vi "SensorcolorV2.vi"() -> ()   [LabVIEW 2017]
panel:
  in  "Guardar en:":path
  out "Sin Filtro":dbl format="%.2f"
  out "Azul":dbl
  out "Verde":dbl format="%.2f"
  out "Rojo":dbl format="%.2f"
  in  "Frecuencia 1":bool=TRUE
  in  "Frecuencia 2":bool
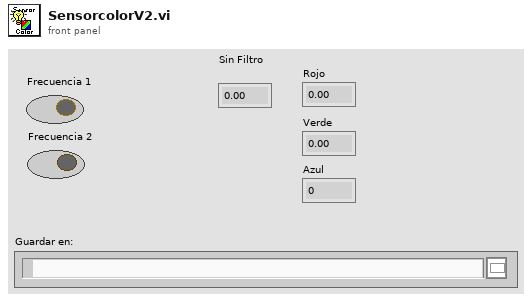
[diagram p1: front panel]
types:
  T1 = enum16{"open", "open or create", "create or replace", "create", "open (read-only)"}
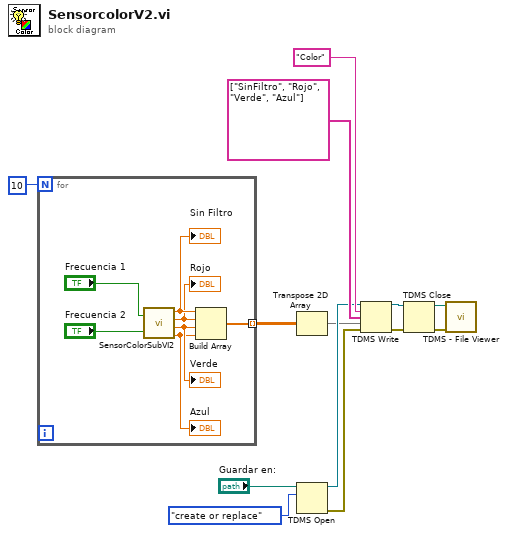
[diagram p0: block diagram]
diagram:
  n1 = for {
    N: 10 -> [_]
    tunnel: [w20] -> w4 mode=indexing
    n2 = call "SensorColorSubVI2.vi"("Frecuencia 1"="Frecuencia 1", "Frecuencia in"="Frecuencia 2") -> ("Sin Filtro"=w17:dbl, "Rojo"=w16:dbl, "Verde"=w15:dbl, "Azul"=w14:dbl)
    "Sin Filtro" <- w17
    "Rojo" <- w16
    "Verde" <- w15
    "Azul" <- w14
    n3 = Build Array(w17, w16, w15, w14) -> (w20:dbl[])
  }
  n4 = Transpose 2D Array(2D array=w4) -> (transposed array=w1:dbl[][])
  n5 = TDMS Open(10:T1."create or replace" ("operation (0:open)"), 11:"Guardar en:") -> (0:w10:errorcluster, 3:w7:refnum<k34>)  [unwired: 5 in]
  n6 = TDMS Write(0:w7, 5:"Color" ("group name in (Untitled)"), 7:string[] ["SinFiltro", "Rojo", "Verde", "Azul"] ("channel name(s) in (Untitled)"), 9:w1, 11:w10) -> (4:w8:refnum<k34>, 15:w9:errorcluster)  [unwired: 1 in, 2 out]
  n7 = TDMS Close(8:w9, 11:w8) -> (0:w6:errorcluster, 3:w5:path)
  n8 = call <vilib>:"TDMS - File Viewer.vi"("error in (no error)"=w6, "file path"=w5) -> ()  [unwired: 4 in, 2 out]
